vi "GetControlSubPanelVI.vi"(8 "error in (no error)":errorcluster, 10 "SubPanelName":string="SubPanel", 11 "CtlLookup In":T1) -> (0 "error out":errorcluster, 1 "VI out":refnum<vi>, 2 "SubPanelRef":refnum<vi>, 3 "CtlLookup Out":T1)   [LabVIEW 2020, in "CtlReferences_API.lvlib"]
doc: "This VI gets the reference to subpanel, and associated VI"
uses:
  CtlReferences_API.lvlib
  TypeDefs/CtlLookup.ctl
  CtlReferences.lvclass
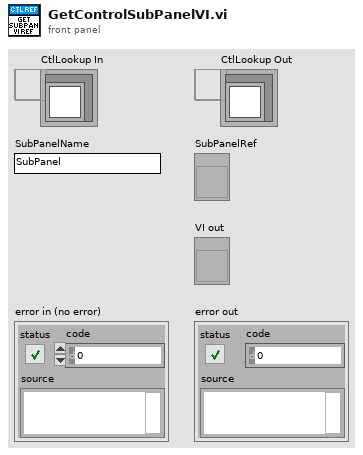
[diagram p1: front panel]
types:
  T1 = typedef "CtlReferences.lvlib/CtlReferences.lvclass/CtlLookup.ctl" = refnum<data-value>
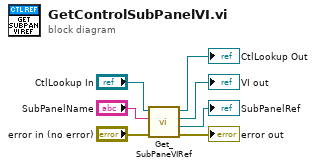
[diagram p0: block diagram]
diagram:
  n1 = call "Get_SubPaneVIRef.vi"("error in (no error)"="error in (no error)", "SubPanelName"="SubPanelName", "CtlLookup In"="CtlLookup In") -> ("error out"=→"error out":errorcluster, "SubPanelRef"=→"SubPanelRef":refnum<vi>, "VI out"=→"VI out":refnum<vi>, "CtlLookup Out"=→"CtlLookup Out":T1)  [unwired: 5 in]
